vi "Email_Attachment_Plot.vi"(1 "X axis name":string, 2 "Y axis name":string, 3 "XY Graph":cluster{dbl[], dbl[]}[](graph), 4 "Series Names":string[](array[string]), 5 "message":string, 6 "subject ([No Subject])":string="[No Subject]") -> ()   [LabVIEW 2010]
uses:
  Email_transfer_global.vi
panel:
  out "Plotted":string
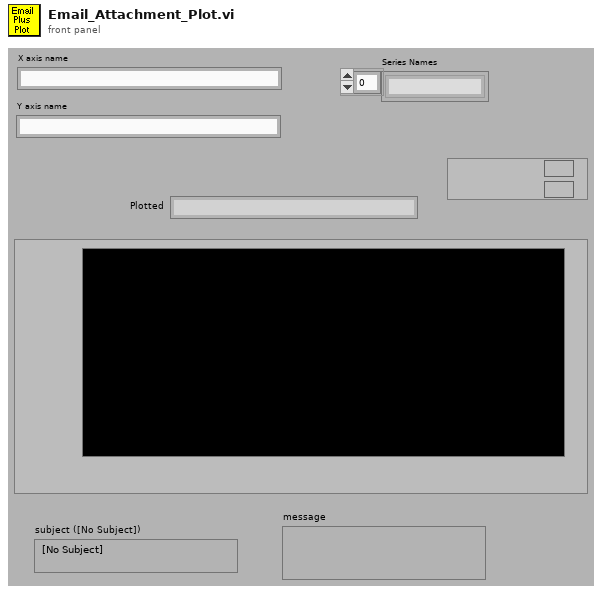
[diagram p1: front panel]
types:
  T1 = cluster{"path":path, "data":string, "binary":bool, "MIME content-type \n(application/octet-stream)":string}[]
  T2 = cluster{"path":path, "data":string, "binary":bool, "MIME content-type \n(application/octet-stream)":string}
  T3 = typedef "LVRectTypeDef.ctl" = cluster{"left":i16, "top":i16, "right":i16, "bottom":i16}
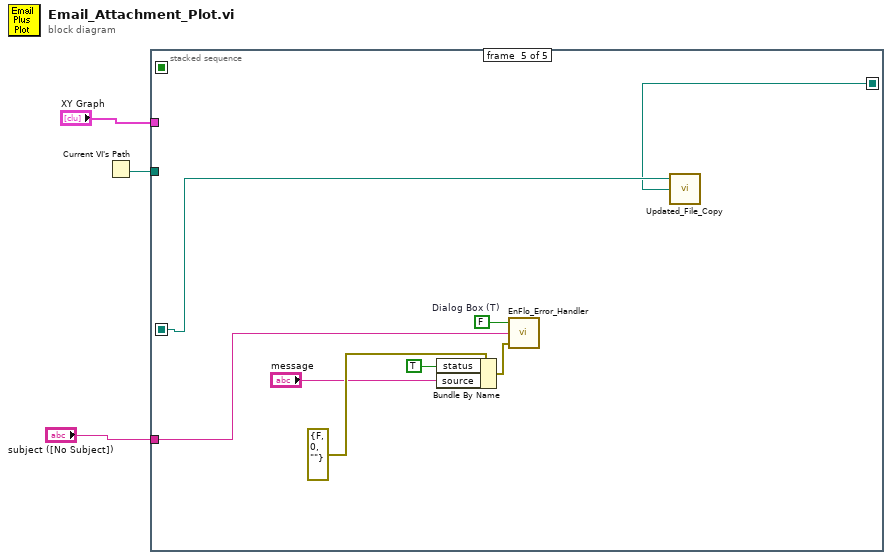
[diagram p0: block diagram]
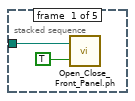
[diagram p2: hidden frame]
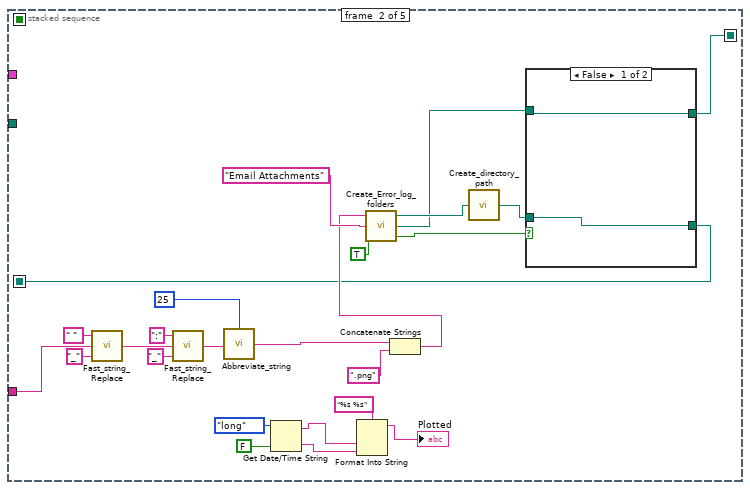
[diagram p3: hidden frame]
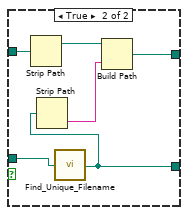
[diagram p4: hidden frame]
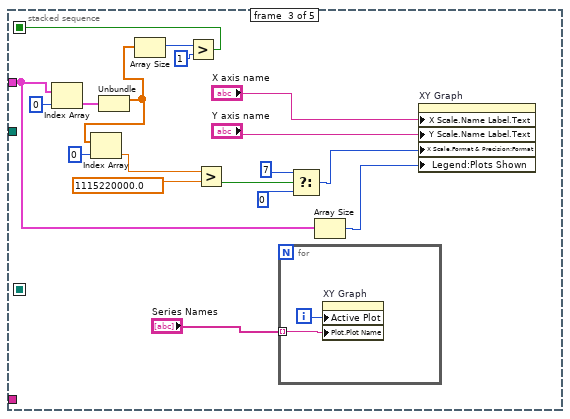
[diagram p5: hidden frame]
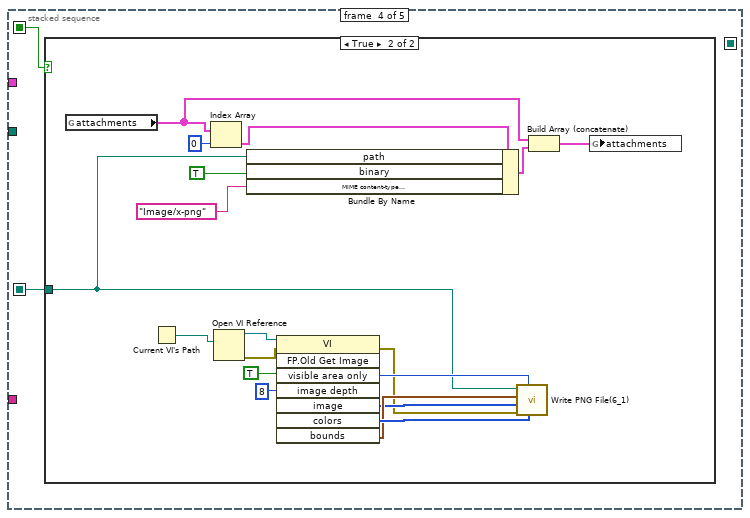
[diagram p6: hidden frame]
diagram:
  n1 = Current VI's Path() -> (path=w1:path)
  n2 = stacked-sequence {
    seq-local: [_ w11 _ _ _] -> [_ _ _ w60 w79]
    seq-local: [_ _ w39 _ _] -> [_ _ _ w59 _]
    seq-local: [_ w6 _ _ _] -> [_ _ _ _ w78]
    tunnel: "subject ([No Subject])" -> [_ w19 _ _ w85]
    tunnel: "XY Graph" -> [_ _ w44 _ _]
    tunnel: w1 -> [w5 _ _ _ _]
    frame #0 {
      n3 = call "Open_Close_Front_Panel.ph.vi"("Front Panel Window:Open"=TRUE, "VI path"=w5) -> ()  [unwired: 2 out]
    }
    frame #1 {
      n4 = call "Fast_string_Replace.vi"("Replace match with:"="_", "Input String"=w19, "regular expression"=" ") -> ("Output String"=w18:string)  [unwired: 2 out]
      n5 = call "Fast_string_Replace.vi"("Replace match with:"="_", "Input String"=w18, "regular expression"=":") -> ("Output String"=w17:string)  [unwired: 2 out]
      n6 = call "Abbreviate_string.vi"("Input String"=w17, "Max String Length"=25 ("length (rest)")) -> ("Output String"=w15:string)
      n7 = Get Date/Time String(date format (0)=enum16{"short", "long", "abbreviated"}."long", want seconds? (F)=FALSE) -> (date string=w27:string, time string=w26:string)  [unwired: 1 out]
      n8 = Format Into String(format string="%s %s", w27, w26) -> (resulting string=→"Plotted":string)  [unwired: 2 in, 1 out]
      n9 = Concatenate Strings(w15, ".png" ("string")) -> (w13:string)
      n10 = call "Create_Error_log_folders.vi"("Per Day Log File?"=TRUE, "Log Folder"="Email Attachments" ("name or relative path"), "Log Filename"=w13) -> ("exists?"=w12:bool, "Server copy Location"=w7:path, "Local Log File"=w10:path)
      n11 = call "Create_directory_path.vi"("Path name"=w10) -> ("Path name Out"=w9:path)
      n12 = case shown="False" w12 {
        tunnel: w9 -> [w32 w38]
        tunnel: [w32 w37] -> w11
        tunnel: w7 -> [w31 w36]
        tunnel: [w31 w33] -> w6
        frame False {
        }
        frame True {
          n13 = Strip Path(path=w36) -> (stripped path=w35:path)  [unwired: 1 out]
          n14 = call "Find_Unique_Filename.vi"("Path In"=w38) -> ("Unique Path Out"=w37:path)  [unwired: 2 in]
          n15 = Strip Path(path=w37) -> (name=w34:string)  [unwired: 1 out]
          n16 = Build Path(base path=w35, name or relative path=w34) -> (appended path=w33:path)
        }
      }
    }
    frame #2 {
      n17 = Index Array(array=w44, index=0) -> (element=w47:cluster{dbl[], dbl[]})
      n18 = Unbundle(w47) -> (w40:dbl[])  [unwired: 1 out]
      n19 = Index Array(array=w40, index=0) -> (element=w45:dbl)
      n20 = Array Size(array=w40) -> (size(s)=w41:i32)
      n21 = Greater?(x=w41, y=1) -> (0:w39:bool)
      n22 = Greater?(x=w45, y=1115220000.0) -> (0:w53:bool)
      n23 = for {
        tunnel: "Series Names" -> [w57] mode=indexing
        i -> [w58]
        n24 = property on="XY Graph" class="XYGraph (strict)"("Active Plot"=w58, "Plot.Plot Name"=w57) -> ()  [unwired: 2 in, 2 out]
      }
      n25 = Select(t=u8 7 ("Write Attribute"), s=w53, f=u8 0 ("Write Attribute")) -> (s? t:f=w49:u8)
      n26 = Array Size(array=w44) -> (size(s)=w43:i32)
      n27 = property on="XY Graph" class="XYGraph (strict)"("X Scale.Name Label.Text"="X axis name", "Y Scale.Name Label.Text"="Y axis name", "X Scale.Format & Precision:Format"=w49, "Legend:Plots Shown"=w43) -> ()  [unwired: 2 in, 2 out]
    }
    frame #3 {
      n28 = case shown="True" w59 {
        tunnel: w60 -> [_ w63]
        frame False {
        }
        frame True {
          w77 = 8 ("image depth")
          n29 = global read "Email_transfer_global.vi" "attachments"() -> (w66:T1)
          n30 = Current VI's Path() -> (path=w69:path)
          n31 = Index Array(array=w66, index=0) -> (element=w67:T2)
          n32 = Open VI Reference(vi path=w69) -> (vi reference=w70:refnum<vi>, error out=w71:errorcluster)  [unwired: 1 in, 4 out]
          n33 = Bundle By Name(cluster=w67, "path"=w63, "binary"=TRUE, "MIME content-type \n(application/octet-stream)"="Image/x-png" ("MIME content-type \n(application/octet-stream)")) -> (w64:T2)
          n34 = invoke class="VI" method="FP.Old Get Image"(reference=w70, error in=w71, "visible area only"=TRUE, "image depth"=w77) -> (error out=w73:errorcluster, "image"=w74:u8[], "colors"=w76:u32[], "bounds"=w75:T3)  [unwired: 4 in, 4 out]
          n35 = call <vilib>:"Write PNG File(6_1).vi"("color table"=w76, "depth"=w77, "error in (no error)"=w73, "flattened image data"=w74, "rect"=w75, "path to PNG file"=w63) -> ()  [unwired: 6 out]
          n36 = Build Array (concatenate)(w66, w64) -> (w65:T1)
          n37 = global write "Email_transfer_global.vi" "attachments"(w65) -> ()
        }
      }
    }
    frame #4 {
      w80 = FALSE  # Dialog Box (T)
      n38 = Bundle By Name(cluster=errorcluster {"status"=FALSE, "code"=0, "source"=""} ("error in (no error)"), "status"=TRUE, "source"="message") -> (w83:errorcluster)
      n39 = call "EnFlo_Error_Handler.vi"("error in (no error)"=w83, "Error Type"=w85, "Dialog Box (T)"=w80) -> ()  [unwired: 3 out]
      n40 = call "Updated_File_Copy.vi"("Target Path"=w78, "Source Path"=w79) -> ()  [unwired: 2 out]
    }
  }
